vi "Update Axis State.vi"(7 "Axis Deadband":dbl=0.15, 8 "error in (no error)":errorcluster, 10 "Axes":dbl[](array[numeric]), 11 "Joystick in":refnum<class "Joystick.lvclass">) -> (0 "error out":errorcluster, 3 "Joystick out":refnum<class "Joystick.lvclass">)   [LabVIEW 2014, in "Joystick.lvlib" / "Joystick.lvclass"]
uses:
  Joystick.lvclass
  Joystick.lvclass/Joystick.ctl
  Axis State.ctl
  Button State.ctl
  Joystick.lvlib
panel:
  in  "Button Threshold":dbl=0.5
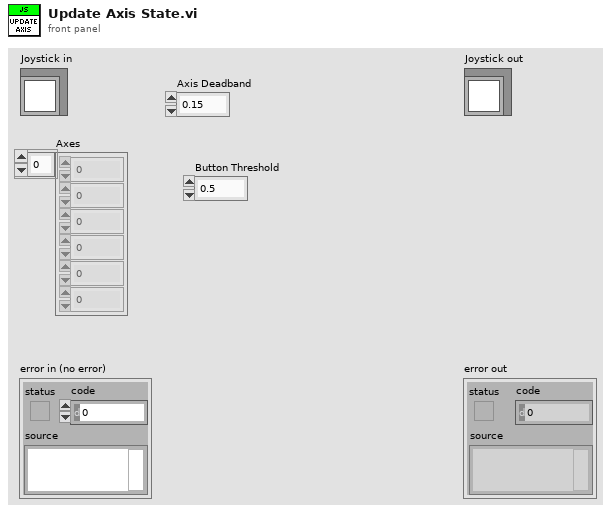
[diagram p1: front panel]
types:
  T1 = typedef "Joystick.lvlib/Joystick.lvclass/Axis State.ctl" = cluster{"Instance Name":string, "Deadband":dbl, "Value":dbl, "At Home":bool, "Postive Axis Button State":T2, "Negative Axis Button State":T2, "Home Axis Button State":T2}
  T2 = typedef "Joystick.lvlib/Joystick.lvclass/Button State.ctl" = cluster{"Pressed":bool, "Instance Name":string, "Toggled":bool, "Just Changed":bool}
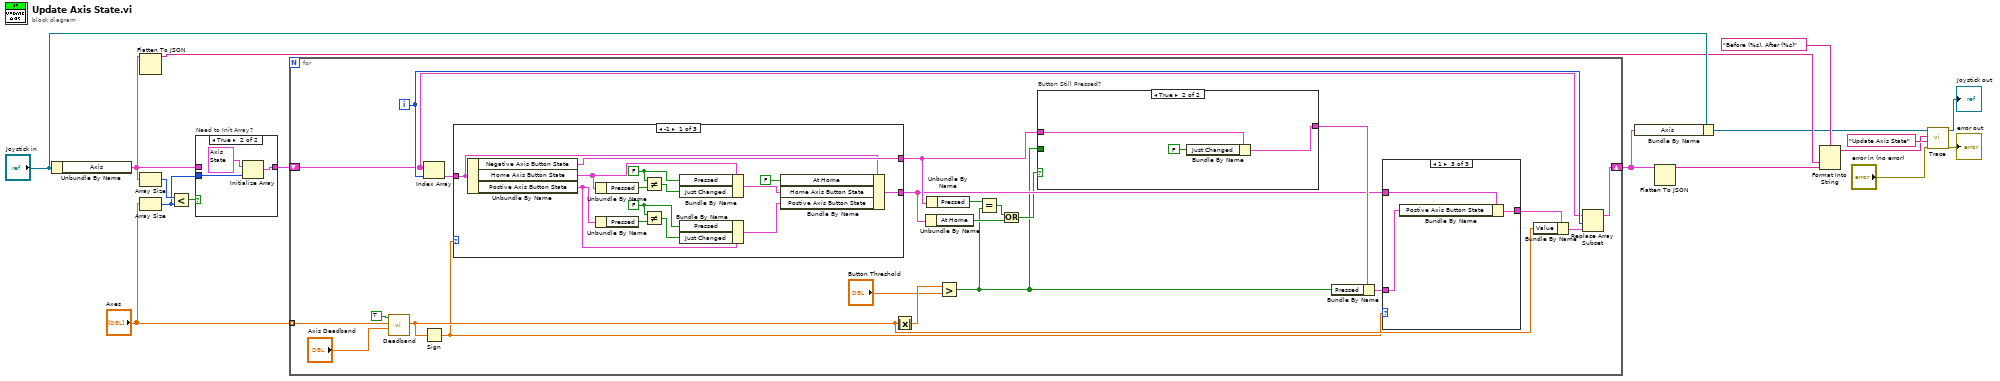
[diagram p0: block diagram]
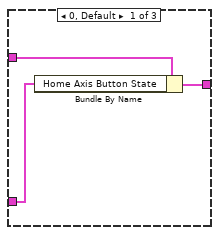
[diagram p3: hidden frame]
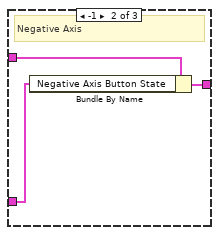
[diagram p4: hidden frame]
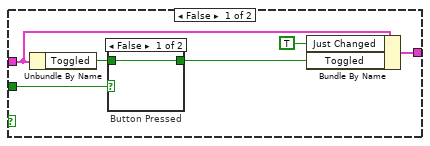
[diagram p5: hidden frame]
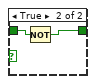
[diagram p6: hidden frame]
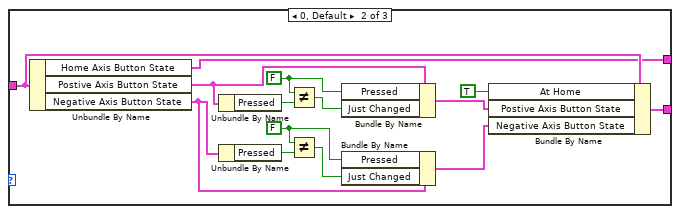
[diagram p7: hidden frame]
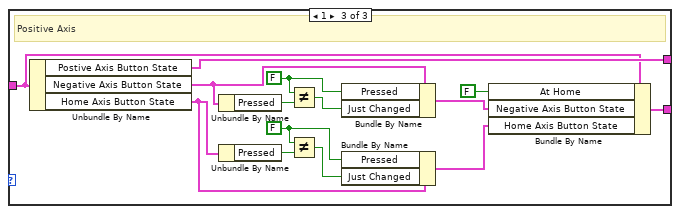
[diagram p8: hidden frame]
diagram:
  n1 = Unbundle By Name("Joystick in") -> ("Axis"=w3:T1[])
  n2 = Flatten To JSON(anything=w3) -> (JSON string=w11:string)  [unwired: 2 in, 1 out]
  n3 = Array Size(array=w3) -> (size(s)=w5:i32)
  n4 = Array Size(array="Axes") -> (size(s)=w1:i32)
  n5 = Less?(x=w5, y=w1) -> (x < y?=w4:bool)
  n6 = case "Need to Init Array?" shown="True" w4 {
    tunnel: w3 -> [w18 _]
    tunnel: [w18 w19] -> w2
    tunnel: w1 -> [_ w21]
    frame False {
    }
    frame True {
      n7 = Initialize Array(T1 {"Instance Name"="", "Deadband"=0.0, "Value"=0.0, "At Home"=FALSE, "Postive Axis Button State"={"Pressed"=FALSE, "Instance Name"="", "Toggled"=FALSE, "Just Changed"=FALSE}, "Negative Axis Button State"={"Pressed"=FALSE, "Instance Name"="", "Toggled"=FALSE, "Just Changed"=FALSE}, "Home Axis Button State"={"Pressed"=FALSE, "Instance Name"="", "Toggled"=FALSE, "Just Changed"=FALSE}} ("Axis State"), w21) -> (w19:T1[])
    }
  }
  n8 = for {
    tunnel: "Axes" -> [w39] mode=indexing
    shift-right: [w42] -> w9
    shift-left: w2 -> [w41]
    i -> [w43]
    n9 = call "Deadband.vi"("Deadband"="Axis Deadband", "Before Deadband"=w39, "Expand Range"=TRUE) -> ("After Deadband"=w34:dbl)  [unwired: 8 in]
    n10 = Index Array(array=w41, index=w43) -> (element=w33:T1)
    n11 = Sign(1:w34) -> (0:w30:dbl)
    n12 = case shown="-1" w30 {
      tunnel: w33 -> [w77 w90 w105]
      tunnel: [w78 w89 w106] -> w31
      tunnel: [w76 w92 w104] -> w26
      frame -1 {
        w65 = FALSE ("x")
        w71 = FALSE ("x")
        n13 = Unbundle By Name(w77) -> ("Negative Axis Button State"=w78:T2, "Home Axis Button State"=w74:T2, "Postive Axis Button State"=w69:T2)
        n14 = Unbundle By Name(w74) -> ("Pressed"=w73:bool)
        n15 = Unbundle By Name(w69) -> ("Pressed"=w68:bool)
        n16 = Not Equal?(x=w71, y=w73) -> (x != y?=w70:bool)
        n17 = Not Equal?(x=w65, y=w68) -> (x != y?=w66:bool)
        n18 = Bundle By Name(cluster=w74, "Pressed"=w71, "Just Changed"=w70) -> (w72:T2)
        n19 = Bundle By Name(cluster=w69, "Pressed"=w65, "Just Changed"=w66) -> (w67:T2)
        n20 = Bundle By Name(cluster=w77, "At Home"=FALSE, "Home Axis Button State"=w72, "Postive Axis Button State"=w67) -> (w76:T1)
      }
      frame 0, Default {
        w80 = FALSE ("x")
        w85 = FALSE ("x")
        n21 = Unbundle By Name(w90) -> ("Home Axis Button State"=w89:T2, "Postive Axis Button State"=w88:T2, "Negative Axis Button State"=w83:T2)
        n22 = Unbundle By Name(w88) -> ("Pressed"=w87:bool)
        n23 = Unbundle By Name(w83) -> ("Pressed"=w82:bool)
        n24 = Not Equal?(x=w85, y=w87) -> (x != y?=w84:bool)
        n25 = Not Equal?(x=w80, y=w82) -> (x != y?=w79:bool)
        n26 = Bundle By Name(cluster=w88, "Pressed"=w85, "Just Changed"=w84) -> (w86:T2)
        n27 = Bundle By Name(cluster=w83, "Pressed"=w80, "Just Changed"=w79) -> (w81:T2)
        n28 = Bundle By Name(cluster=w90, "At Home"=TRUE, "Postive Axis Button State"=w86, "Negative Axis Button State"=w81) -> (w92:T1)
      }
      frame 1 {
        w94 = FALSE ("Pressed")
        w98 = FALSE ("Pressed")
        # "Positive Axis"
        n29 = Unbundle By Name(w105) -> ("Postive Axis Button State"=w106:T2, "Negative Axis Button State"=w100:T2, "Home Axis Button State"=w97:T2)
        n30 = Unbundle By Name(w100) -> ("Pressed"=w99:bool)
        n31 = Unbundle By Name(w97) -> ("Pressed"=w96:bool)
        n32 = Not Equal?(x=w98, y=w99) -> (x != y?=w95:bool)
        n33 = Not Equal?(x=w94, y=w96) -> (x != y?=w93:bool)
        n34 = Bundle By Name(cluster=w100, "Pressed"=w98, "Just Changed"=w95) -> (w102:T2)
        n35 = Bundle By Name(cluster=w97, "Pressed"=w94, "Just Changed"=w93) -> (w101:T2)
        n36 = Bundle By Name(cluster=w105, "At Home"=FALSE, "Negative Axis Button State"=w102, "Home Axis Button State"=w101) -> (w104:T1)
      }
    }
    n37 = Absolute Value(x=w34) -> (abs(x)=w36:dbl)
    n38 = Unbundle By Name(w26) -> ("At Home"=w25:bool)
    n39 = Unbundle By Name(w31) -> ("Pressed"=w32:bool)
    n40 = Greater?(x=w36, y="Button Threshold") -> (0:w22:bool)
    n41 = Equal?(x=w32, y=w22) -> (x = y?=w27:bool)
    n42 = Or(x=w27, y=w25) -> (x .or. y?=w24:bool)
    n43 = case "Button Still Pressed?" shown="True" w24 {
      tunnel: w31 -> [w57 w64]
      tunnel: [w54 w63] -> w29
      tunnel: w22 -> [w53 _]
      frame False {
        n44 = Unbundle By Name(w57) -> ("Toggled"=w58:bool)
        n45 = case "Button Pressed" shown="False" w53 {
          tunnel: w58 -> [w59 w61]
          tunnel: [w59 w60] -> w55
          frame False {
          }
          frame True {
            n46 = Not(x=w61) -> (.not. x?=w60:bool)
          }
        }
        n47 = Bundle By Name(cluster=w57, "Just Changed"=TRUE, "Toggled"=w55) -> (w54:T2)
      }
      frame True {
        n48 = Bundle By Name(cluster=w64, "Just Changed"=FALSE) -> (w63:T2)
      }
    }
    n49 = Bundle By Name(cluster=w29, "Pressed"=w22) -> (w23:T2)
    n50 = case shown="1" w30 {
      tunnel: w23 -> [w44 w47 w51]
      tunnel: w26 -> [w46 w49 w52]
      tunnel: [w45 w48 w50] -> w28
      frame 0, Default {
        n51 = Bundle By Name(cluster=w46, "Home Axis Button State"=w44) -> (w45:T1)
      }
      frame -1 {
        # "Negative Axis"
        n52 = Bundle By Name(cluster=w49, "Negative Axis Button State"=w47) -> (w48:T1)
      }
      frame 1 {
        n53 = Bundle By Name(cluster=w52, "Postive Axis Button State"=w51) -> (w50:T1)
      }
    }
    n54 = Bundle By Name(cluster=w28, "Value"=w34) -> (w40:T1)
    n55 = Replace Array Subset(array=w41, new element=w40, index=w43) -> (w42:T1[])
  }
  n56 = Bundle By Name(cluster="Joystick in", "Axis"=w9) -> (w10:refnum<class "Joystick.lvclass">)
  n57 = Flatten To JSON(anything=w9) -> (JSON string=w8:string)  [unwired: 2 in, 1 out]
  n58 = Format Into String(format string="Before (%s), After (%s)", w11, w8) -> (resulting string=w7:string)  [unwired: 2 in, 1 out]
  n59 = call-dynamic "Trace.vi"("error in (no error)"="error in (no error)", "System Message"=w7, "System Action"="Update Axis State", "System Actor in"=w10) -> ("error out"=→"error out":errorcluster, "System Actor out"=→"Joystick out":refnum<class "Joystick.lvclass">)  [unwired: 6 in]
